vi "Stop Video.vi"(5 "Frame Rate(Hz)":cluster{"AVI FR":i32, "Camera Fr":u16}={"AVI FR"=30, "Camera Fr"=0} {"AVI FR" min=2 max=3000 step=1}, 6 "Save Movie?":bool, 7 "Trigger Type":enum16{"Internal", "External"}(ring)=enum."External", 8 "error in":errorcluster, 9 "Frame Buffers In":T2[](array[typedef]), 10 "Avi Refnum":T1, 11 "IMAQ Session In":refnum<k11>) -> (0 "error out":errorcluster, 3 "Buffer Number":i32)   [LabVIEW 2013]
uses:
  <vilib>/vision/Image Controls.llb/IMAQ Image.ctl
  <vilib>/vision/Avi1.llb/AviRefnum.ctl
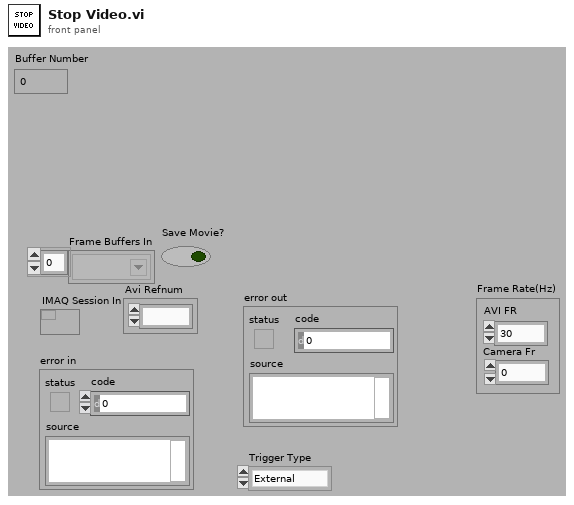
[diagram p1: front panel]
types:
  T1 = typedef "AviRefnum.ctl" = refnum<k1>
  T2 = typedef "IMAQ Image.ctl" = refnum<image>
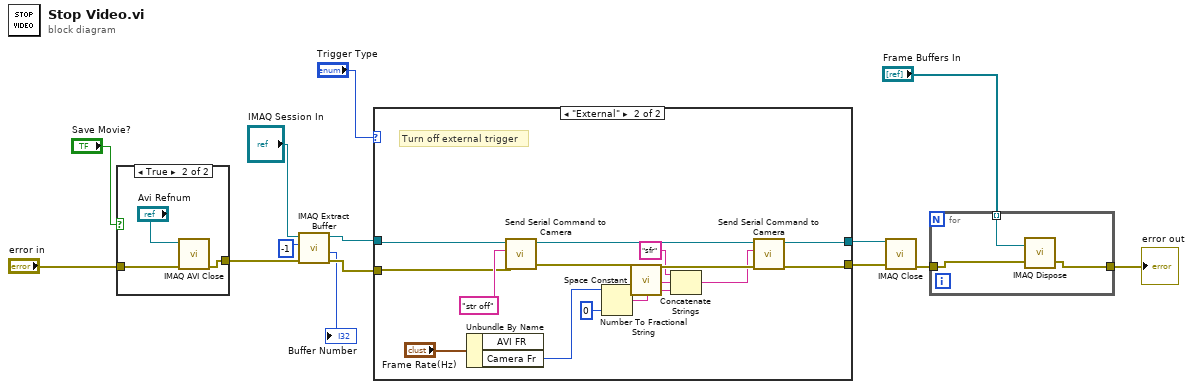
[diagram p0: block diagram]
diagram:
  n1 = case shown="True" "Save Movie?" {
    tunnel: "error in" -> [w15 w18]
    tunnel: [w15 w16] -> w8
    frame False {
    }
    frame True {
      n2 = call "IMAQ AVI Close"("error in (no error)"=w18, "Avi Refnum"="Avi Refnum") -> ("error out"=w16:errorcluster)  [unwired: 9 in]
    }
  }
  n3 = call <vilib>:"IMAQ Extract Buffer.vi"("error in (no error)"=w8, "Buffer to extract"=-1, "IMAQ Session In"="IMAQ Session In") -> ("error out"=w5:errorcluster, "Buffer Number"=→"Buffer Number":i32, "IMAQ Session Out"=w6:refnum<k11>)  [unwired: 3 in, 3 out]
  n4 = case shown="\"External\"" "Trigger Type" {
    tunnel: w6 -> [w20 w24]
    tunnel: w5 -> [w19 w23]
    tunnel: [w19 w21] -> w3
    tunnel: [w20 w22] -> w4
    frame "Internal", Default {
    }
    frame "External" {
      # "Turn off external trigger"
      n5 = Unbundle By Name("Frame Rate(Hz)") -> ("Camera Fr"=w25:u16)  [unwired: 1 out]
      n6 = call "Send Serial Command to Camera.vi"("error in (no error)"=w23, "String to write"="str off", "IMAQ Session In"=w24) -> ("error out"=w33:errorcluster, "IMAQ Session Out"=w32:refnum<k11>)  [unwired: 5 in, 2 out]
      n7 = Number To Fractional String(number=w25, precision (6)=i16 0) -> (F-format string=w29:string)  [unwired: 2 in]
      n8 = call <vilib>:"Space Constant.vi"() -> ("String"=w28:string)
      n9 = Concatenate Strings("sfr" ("string"), w28, w29) -> (w31:string)
      n10 = call "Send Serial Command to Camera.vi"("error in (no error)"=w33, "String to write"=w31, "IMAQ Session In"=w32) -> ("error out"=w21:errorcluster, "IMAQ Session Out"=w22:refnum<k11>)  [unwired: 5 in, 2 out]
    }
  }
  n11 = call <vilib>:"IMAQ Close.vi"("error in (no error)"=w3, "IMAQ Session In"=w4) -> ("error out"=w12:errorcluster)  [unwired: 9 in]
  n12 = for {
    tunnel: [w37] -> w10
    tunnel: w12 -> [w35]
    tunnel: "Frame Buffers In" -> [w36] mode=indexing
    n13 = call "IMAQ Dispose"("Image"=w36, "error in (no error)"=w35) -> ("error out"=w37:errorcluster)  [unwired: 4 in]
  }
  "error out" <- w10
